vi "Calibrate.vi"(8 "RF  FREQUENCY MHz":dbl=1000.0 min=55.0 max=14000.0 step=1.0 format="%_11g", 10 "CalData":string[][](array[string]), 11 "RF Power In":dbl) -> (0 "Unleveled":bool, 2 "cal level":string, 3 "Power Out Display":dbl)   [LabVIEW 2012]
panel:
  out "HighCoerc":dbl
  out "LowCoerc":dbl
  out "LevTR":string
  out "LevTL":string
  out "LevBL":string
  out "LevBR":string
  # "4 Cal Levels surrounding desired\nfrequency and power"
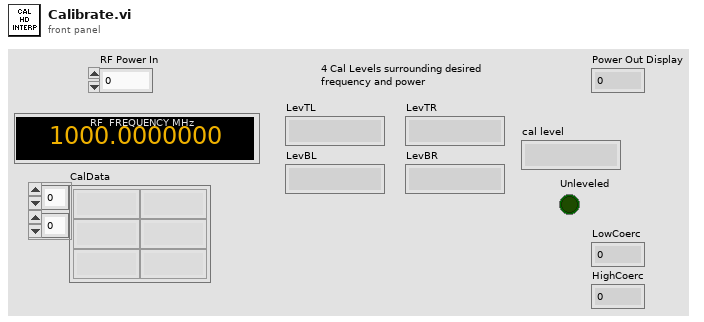
[diagram p1: front panel]
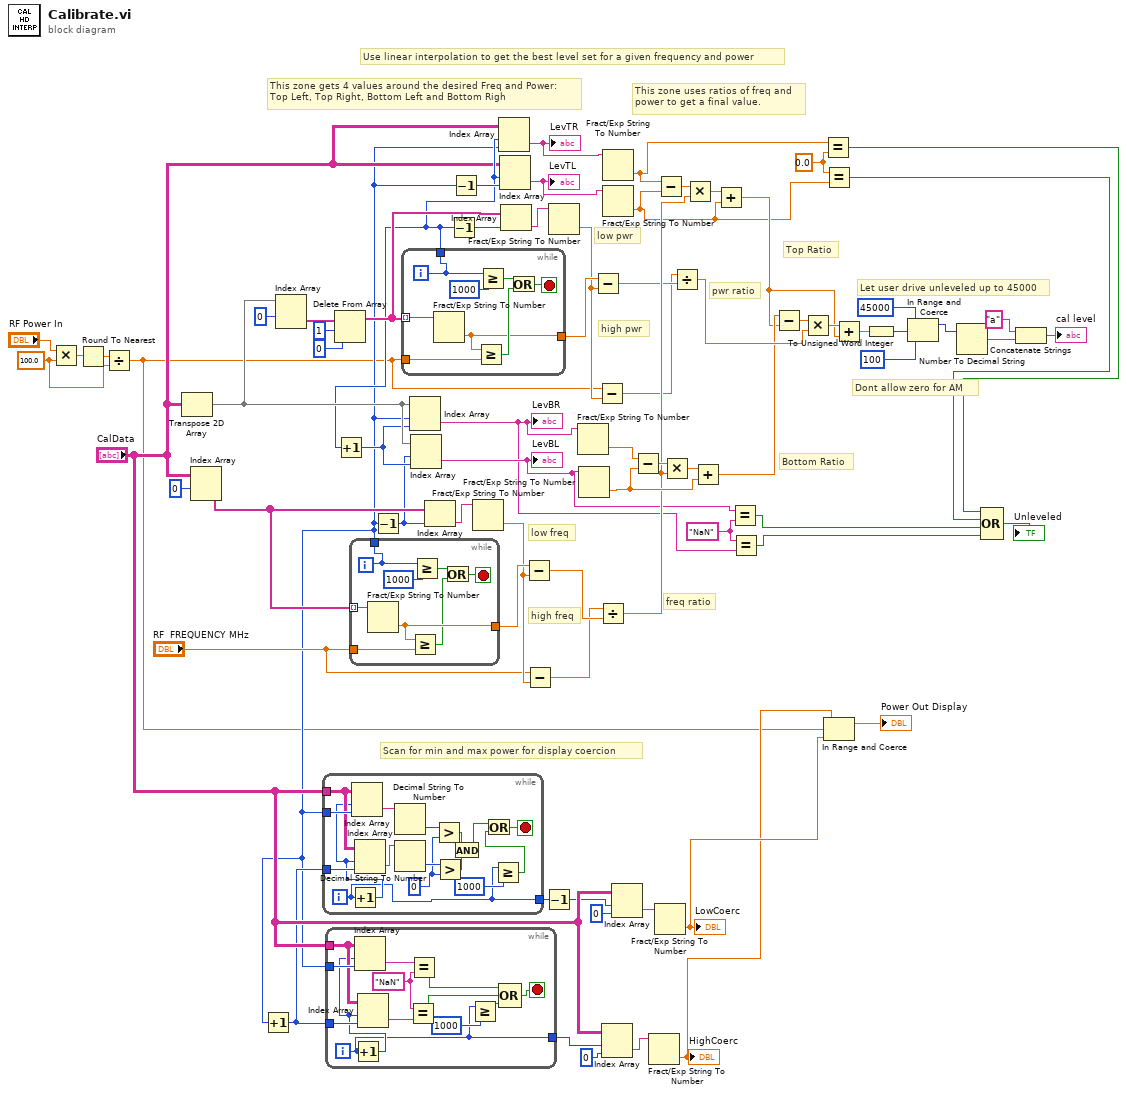
[diagram p0: block diagram]
diagram:
  w3 = 100.0 ("y")
  w10 = 0.0 ("x")
  w30 = "NaN" ("y")
  # "Dont allow zero for AM"
  # "Let user drive unleveled up to 45000"
  # "Scan for min and max power for display coercion"
  # "Bottom Ratio"
  # "Top Ratio"
  # "pwr ratio"
  # "freq ratio"
  # "high pwr"
  # "low pwr"
  # "high freq"
  # "low freq"
  # "Use linear interpolation to get the best level set for a given frequency and power"
  # "This zone uses ratios of freq and\npower to get a final value."
  # "This zone gets 4 values around the desired Freq and Power:\nTop Left, Top Right, Bottom Left and Bottom Righ"
  n1 = Multiply(x="RF Power In", y=w3) -> (x*y=w5:dbl)
  n2 = Round To Nearest(number=w5) -> (nearest integer value=w4:dbl)
  n3 = Divide(x=w4, y=w3) -> (x/y=w1:dbl)
  n4 = Transpose 2D Array(2D array="CalData") -> (transposed array=w66:string[][])
  n5 = Index Array(array="CalData", index (row)=0) -> (element=w74:string[])  [unwired: 1 in]
  n6 = Index Array(array=w66, index (row)=0) -> (element=w71:string[])  [unwired: 1 in]
  n7 = Delete From Array(array=w71, length=1, index=0) -> (array with subset deleted=w67:string[])  [unwired: 1 out]
  n8 = while {
    tunnel: w74 -> [w83] mode=indexing
    tunnel: "RF  FREQUENCY MHz" -> [w82]
    tunnel: [w79] -> w58
    tunnel: [w76] -> w13
    i -> [w76]
    stop <- w81 stop-if-true
    n9 = Fract/Exp String To Number(string=w83) -> (number=w79:dbl)  [unwired: 3 in, 1 out]
    n10 = Greater Or Equal?(x=w79, y=w82) -> (x >= y?=w77:bool)
    n11 = Greater Or Equal?(x=w76, y=1000) -> (x >= y?=w78:bool)
    n12 = Or(x=w78, y=w77) -> (x .or. y?=w81:bool)
  }
  n13 = Increment(x=w13) -> (x+1=w14:i32)
  n14 = while {
    tunnel: w13 -> [w99]
    tunnel: w14 -> [w98]
    tunnel: "CalData" -> [w97]
    tunnel: [w87] -> w12
    i -> [w87]
    stop <- w86 stop-if-true
    w92 = 0 ("y")
    n15 = Increment(x=w87) -> (x+1=w89:i32)
    n16 = Index Array(array=w97, index (row)=w89, index (col)=w99) -> (element=w95:string)
    n17 = Index Array(array=w97, index (row)=w89, index (col)=w98) -> (element=w96:string)
    n18 = Decimal String To Number(string=w95) -> (number=w94:i32)  [unwired: 2 in, 1 out]
    n19 = Decimal String To Number(string=w96) -> (number=w93:i32)  [unwired: 2 in, 1 out]
    n20 = Greater?(x=w94, y=w92) -> (0:w91:bool)
    n21 = Greater?(x=w93, y=w92) -> (0:w90:bool)
    n22 = And(x=w91, y=w90) -> (x .and. y?=w84:bool)
    n23 = Greater Or Equal?(x=w87, y=1000) -> (x >= y?=w85:bool)
    n24 = Or(x=w84, y=w85) -> (x .or. y?=w86:bool)
  }
  n25 = while {
    tunnel: w13 -> [w112]
    tunnel: w14 -> [w111]
    tunnel: "CalData" -> [w110]
    tunnel: [w101] -> w20
    i -> [w101]
    stop <- w109 stop-if-true
    w106 = "NaN" ("x")
    n26 = Increment(x=w101) -> (x+1=w103:i32)
    n27 = Index Array(array=w110, index (row)=w103, index (col)=w112) -> (element=w108:string)
    n28 = Index Array(array=w110, index (row)=w103, index (col)=w111) -> (element=w107:string)
    n29 = Equal?(x=w106, y=w107) -> (x = y?=w105:bool)
    n30 = Equal?(x=w108, y=w106) -> (x = y?=w104:bool)
    n31 = Greater Or Equal?(x=w101, y=1000) -> (x >= y?=w100:bool)
    n32 = Compound Arithmetic op=OR(w104, w105, w100) -> (w109:bool)
  }
  n33 = Decrement(x=w13) -> (x-1=w23:i32)
  n34 = while {
    tunnel: w67 -> [w120] mode=indexing
    tunnel: w1 -> [w119]
    tunnel: [w114] -> w51
    tunnel: [w113] -> w36
    i -> [w113]
    stop <- w118 stop-if-true
    n35 = Fract/Exp String To Number(string=w120) -> (number=w114:dbl)  [unwired: 3 in, 1 out]
    n36 = Greater Or Equal?(x=w114, y=w119) -> (x >= y?=w115:bool)
    n37 = Greater Or Equal?(x=w113, y=1000) -> (x >= y?=w116:bool)
    n38 = Or(x=w116, y=w115) -> (x .or. y?=w118:bool)
  }
  n39 = Increment(x=w36) -> (x+1=w37:i32)
  n40 = Index Array(array=w66, index (row)=w13, index (col)=w37) -> (element=w25:string)
  "LevBR" <- w25
  n41 = Index Array(array=w66, index (row)=w23, index (col)=w37) -> (element=w26:string)
  "LevBL" <- w26
  n42 = Index Array(array=w74, index=w23) -> (element=w73:string)
  n43 = Decrement(x=w36) -> (x-1=w65:i32)
  n44 = Decrement(x=w13) -> (x-1=w52:i32)
  n45 = Fract/Exp String To Number(string=w73) -> (number=w54:dbl)  [unwired: 3 in, 1 out]
  n46 = Index Array(array="CalData", index (row)=w36, index (col)=w13) -> (element=w31:string)
  "LevTR" <- w31
  n47 = Index Array(array="CalData", index (row)=w36, index (col)=w52) -> (element=w29:string)
  "LevTL" <- w29
  n48 = Index Array(array=w67, index=w65) -> (element=w68:string)
  n49 = Subtract(x=w58, y=w54) -> (x-y=w64:dbl)
  n50 = Subtract(x="RF  FREQUENCY MHz", y=w54) -> (x-y=w63:dbl)
  n51 = Decrement(x=w12) -> (x-1=w11:i32)
  n52 = Fract/Exp String To Number(string=w68) -> (number=w49:dbl)  [unwired: 3 in, 1 out]
  n53 = Fract/Exp String To Number(string=w25) -> (number=w56:dbl)  [unwired: 3 in, 1 out]
  n54 = Fract/Exp String To Number(string=w26) -> (number=w57:dbl)  [unwired: 3 in, 1 out]
  n55 = Subtract(x=w51, y=w49) -> (x-y=w50:dbl)
  n56 = Subtract(x=w1, y=w49) -> (x-y=w48:dbl)
  n57 = Divide(x=w63, y=w64) -> (x/y=w55:dbl)
  n58 = Index Array(array="CalData", index (row)=w20, index (col)=0) -> (element=w17:string)
  n59 = Fract/Exp String To Number(string=w31) -> (number=w9:dbl)  [unwired: 3 in, 1 out]
  n60 = Fract/Exp String To Number(string=w29) -> (number=w8:dbl)  [unwired: 3 in, 1 out]
  n61 = Index Array(array="CalData", index (row)=w11, index (col)=0) -> (element=w18:string)
  n62 = Subtract(x=w56, y=w57) -> (x-y=w62:dbl)
  n63 = Fract/Exp String To Number(string=w17) -> (number=w15:dbl)  [unwired: 3 in, 1 out]
  "HighCoerc" <- w15
  n64 = Fract/Exp String To Number(string=w18) -> (number=w16:dbl)  [unwired: 3 in, 1 out]
  "LowCoerc" <- w16
  n65 = Subtract(x=w9, y=w8) -> (x-y=w60:dbl)
  n66 = Multiply(x=w62, y=w55) -> (x*y=w61:dbl)
  n67 = Divide(x=w48, y=w50) -> (x/y=w45:dbl)
  n68 = Multiply(x=w60, y=w55) -> (x*y=w59:dbl)
  n69 = Add(x=w61, y=w57) -> (x+y=w35:dbl)
  n70 = Add(x=w59, y=w8) -> (x+y=w34:dbl)
  n71 = Equal?(x=w26, y=w30) -> (x = y?=w28:bool)
  n72 = Equal?(x=w30, y=w25) -> (x = y?=w27:bool)
  n73 = Subtract(x=w35, y=w34) -> (x-y=w47:dbl)
  n74 = Multiply(x=w47, y=w45) -> (x*y=w46:dbl)
  n75 = Equal?(x=w9, y=w10) -> (x = y?=w6:bool)
  n76 = Equal?(x=w10, y=w8) -> (x = y?=w7:bool)
  n77 = In Range and Coerce(upper limit=w15, x=w1, lower limit=w16) -> (coerced(x)=→"Power Out Display":dbl)  [unwired: 1 out]
  n78 = Add(x=w46, y=w34) -> (x+y=w44:dbl)
  n79 = To Unsigned Word Integer(number=w44) -> (unsigned 16bit integer=w40:u16)
  n80 = In Range and Coerce(upper limit=u16 45000, x=w40, lower limit=u16 100) -> (coerced(x)=w33:u16)  [unwired: 1 out]
  n81 = Number To Decimal String(number=w33) -> (decimal integer string=w43:string)  [unwired: 1 in]
  n82 = Compound Arithmetic op=OR(w6, w7, w28, w27) -> (→"Unleveled":bool)
  n83 = Concatenate Strings("a" ("string"), w43) -> (→"cal level":string)
